vi "Test Bench.vi"() -> ()   [LabVIEW 2018, in "TwinCAT ADS.lvclass"]
uses:
  TwinCAT ADS.lvclass
  Controls/Symbol Information.ctl
  Controls/PLC Type.ctl
  TwinCAT.Ads
panel:
  out "data string":string
  out "output array":u8[](array[numeric])
  out "Value":variant
  out "PLC Type":T1
  out "IsStruct":bool
  out "Symbol Information":T2 {"Type ID" items=["ADST_VOID"=0, "ADST_INT16"=2, "ADST_INT32"=3, "ADST_REAL32"=4, "ADST_REAL64"=5, "ADST_INT8"=16, "ADST_UINT8"=17, "ADST_UINT16"=18, "ADST_UINT32"=19, "ADST_INT64"=20, "ADST_UINT64"=21, "ADST_STRING"=30, "ADST_WSTRING"=31, "ADST_REAL80"=32, "ADST_BIT"=33, "ADST_MAXTYPES"=34, "ADST_BIGTYPE"=65]; "Type Category" items=["Unknown, None"=0, "Primitive"=1, "Alias"=2, "Enum"=3, "Array"=4, "Struct"=5, "FunctionBlock"=6, "Program"=7, "Function"=8, "SubRange"=9, "String"=10, "Bitset"=12, "Pointer"=13, "Union"=14, "Reference"=15, "Interface"=16]}
  out "Out Params":variant[](array[variant])
  out "Return":variant
  out "x-y":dbl format="%^#_6e"
  out "*(type *) &x":u8[](array[numeric])
  out "Byte Stream":u8[](array[numeric])
  # "21.7E-6"
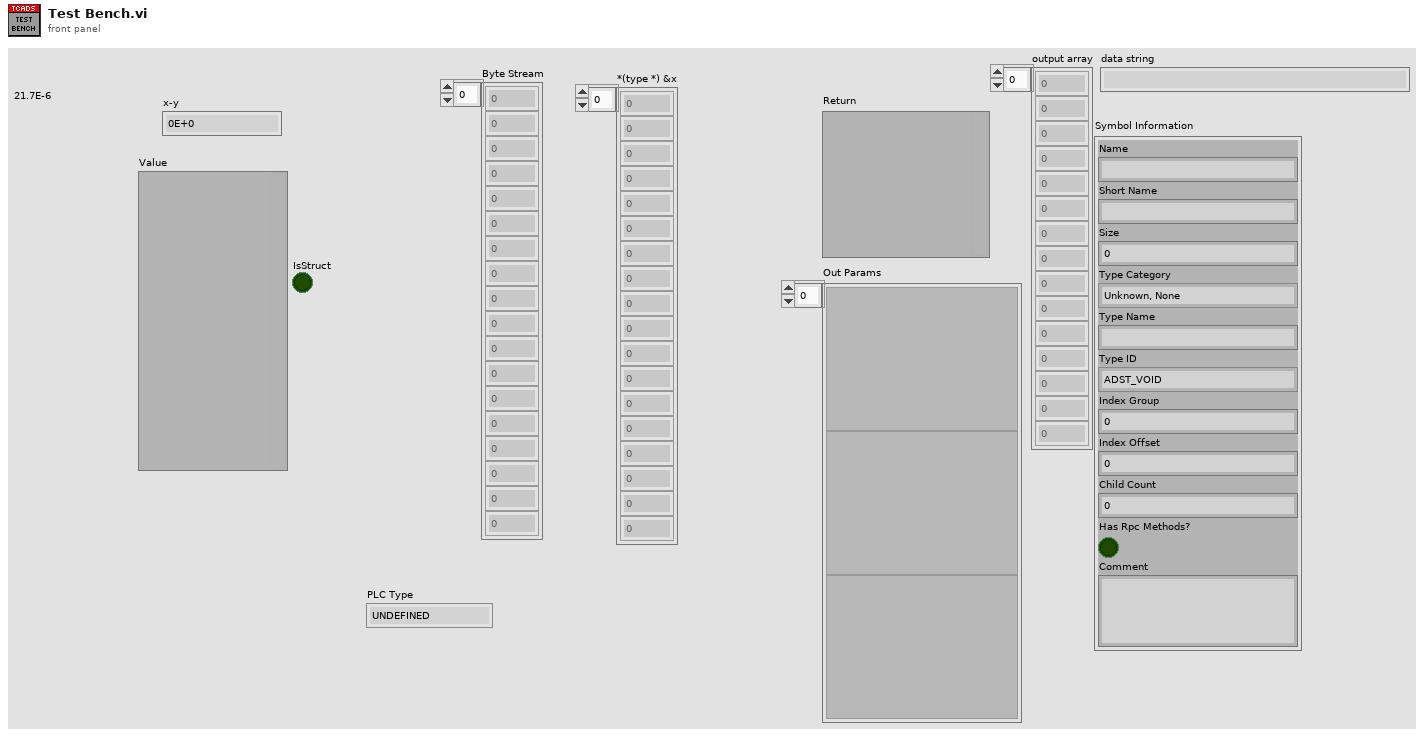
[diagram p1: front panel]
types:
  T1 = typedef "TwinCAT ADS.lvclass/PLC Type.ctl" = enum16{"UNDEFINED", "INT", "DINT", "REAL", "LREAL", "SINT", "BYTE", "UINT", "UDINT", "LINT", "ULINT", "STRING", "WSTRING", "BOOL", "TIME", "LTIME", "DATE", "DT", "TOD", "ARRAY", "JAGGED ARRAY", "STRUCT", "FUNCTION BLOCK", "UNION", "POINTER", "USER DEFINED"}
  T2 = typedef "TwinCAT ADS.lvclass/Symbol Information.ctl" = cluster{"Name":string, "Short Name":string, "Size":i32, "Type Category":i32, "Type Name":string, "Type ID":i32, "Index Group":i64, "Index Offset":i64, "Child Count":i32, "Has Rpc Methods?":bool, "Comment":string}
  T3 = enum16{"big-endian, network order", "native, host order", "little-endian"}
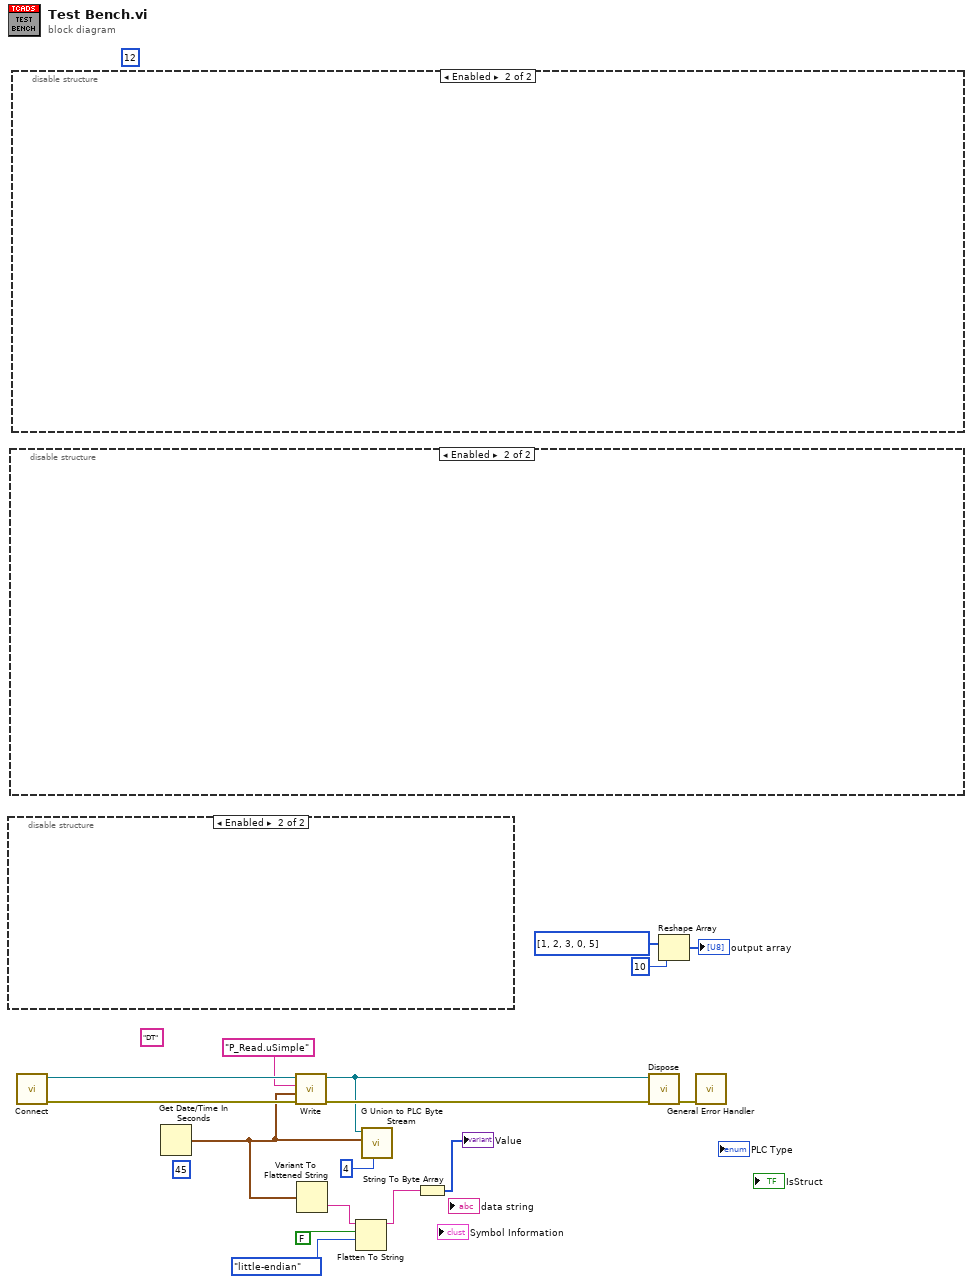
[diagram p0: block diagram]
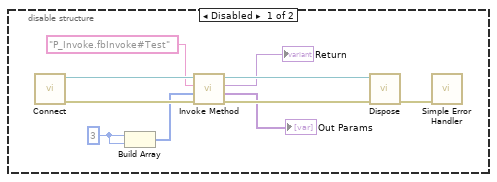
[diagram p2: hidden frame]
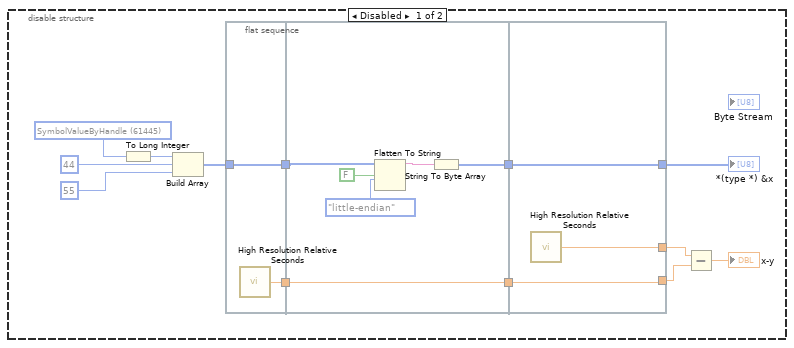
[diagram p3: hidden frame]
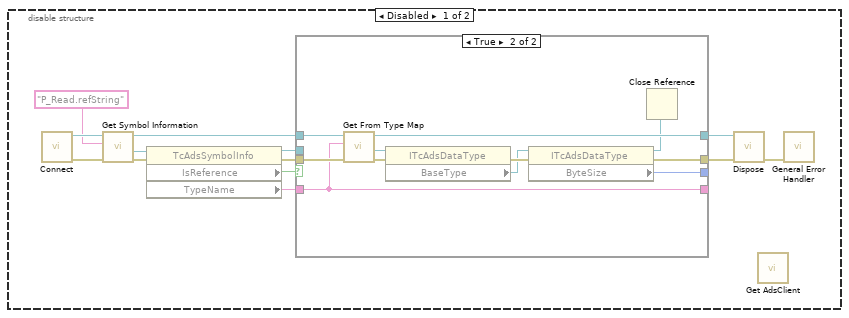
[diagram p4: hidden frame]
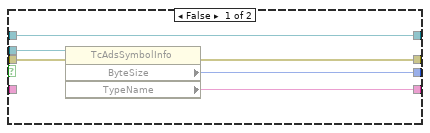
[diagram p5: hidden frame]
diagram:
  (unwired) u8 45 ("new element/subarray")
  (unwired) "DT" ("Type Name")
  (unwired) i16 12
  n1 = disable-structure shown="Enabled" {
    frame Disabled {
      w17 = 3
      n2 = call "Connect.vi"() -> ("error out"=w24:errorcluster, "TwinCAT ADS out"=w25:refnum<class "TwinCAT ADS.lvclass">)  [unwired: 10 in]
      n3 = Build Array(w17, w17) -> (w18:i32[])
      n4 = call "Invoke Method.vi"("error in (no error)"=w24, "In Parameters"=w18, "Function Block#Method"="P_Invoke.fbInvoke#Test", "TwinCAT ADS in"=w25) -> ("error out"=w23:errorcluster, "Out Parameters"=→"Out Params":variant[], "Return"=→"Return":variant, "TwinCAT ADS out"=w22:refnum<class "TwinCAT ADS.lvclass">)  [unwired: 4 in]
      n5 = call "Dispose.vi"("error in (no error)"=w23, "TwinCAT ADS in"=w22) -> ("error out"=w26:errorcluster)  [unwired: 9 in]
      n6 = call <vilib>:"Simple Error Handler.vi"("error in (no error)"=w26) -> ()  [unwired: 4 in, 5 out]
    }
    frame Enabled {
    }
  }
  n7 = disable-structure shown="Enabled" {
    frame Disabled {
      w32 = u32 61445 items=["PlcRWIB"=16384, "PlcRWOB"=16400, "PlcRWMB"=16416, "PlcRWRB"=16432, "PlcRWDB"=16448, "SymbolTable"=61440, "SymbolName"=61441, "SymbolValue"=61442, "SymbolHandleByName"=61443, "SymbolValueByName"=61444, "SymbolValueByHandle"=61445, "SymbolReleaseHandle"=61446, "SymbolInfoByName"=61447, "SymbolVersion"=61448, "SymbolInfoByNameEx"=61449, "SymbolDownload"=61450, "SymbolUpload"=61451, "SymbolUploadInfo"=61452, "SymbolNote"=61456, "IOImageRWIB"=61472, "IOImageRWIX"=61473, "IOImageRWOB"=61488, "IOImageRWOX"=61489, "IOImageClearI"=61504, "IOImageClearO"=61520, "SumCommandRead"=61568, "SumCommandWrite"=61569, "SumCommandReadWrite"=61570, "SumCommandReadEx"=61571, "SumCommandReadEx2"=61572, "SumCommandAddDevNote"=61573, "SumCommandDelDevNote"=61574, "DeviceData"=61696] ("SumCommandRead")
      n8 = To Long Integer(number=w32) -> (32bit integer=w33:i32)
      n9 = Build Array(w33, 44 ("Handle"), 55 ("ByteSize")) -> (w31:i32[])
      n10 = flat-sequence {
        tunnel: w31 -> [w41]
        tunnel: [w41] -> w39
        tunnel: [w40] -> w38
        tunnel: w39 -> [w44]
        tunnel: [w42] -> w37
        tunnel: w38 -> [w47]
        tunnel: [w47] -> w36
        tunnel: [w50] -> w27
        tunnel: w37 -> [w50]
        tunnel: w36 -> [w49]
        tunnel: [w49] -> w29
        tunnel: [w48] -> w30
        frame #0 {
          n11 = call <vilib>:"High Resolution Relative Seconds.vi"() -> ("relative seconds"=w40:dbl)
        }
        frame #1 {
          n12 = Flatten To String(anything=w44, prepend array or string size? (T)=FALSE, byte order (0:big-endian, network order)=T3."little-endian" ("Byte Order (little-endian)")) -> (data string=w43:string)  [unwired: 1 in, 2 out]
          n13 = String To Byte Array(string=w43) -> (unsigned byte array=w42:u8[])
        }
        frame #2 {
          n14 = call <vilib>:"High Resolution Relative Seconds.vi"() -> ("relative seconds"=w48:dbl)
        }
      }
      n15 = Subtract(x=w30, y=w29) -> (x-y=→"x-y":dbl)
      "*(type *) &x" <- w27
    }
    frame Enabled {
    }
  }
  n16 = disable-structure shown="Enabled" {
    frame Disabled {
      n17 = call "Connect.vi"() -> ("error out"=w59:errorcluster, "TwinCAT ADS out"=w60:refnum<class "TwinCAT ADS.lvclass">)  [unwired: 10 in]
      n18 = call "Get Symbol Information.vi"("error in (no error)"=w59, "Symbol Name"="P_Read.refString", "TwinCAT ADS in"=w60) -> ("error out"=w62:errorcluster, ".NET Symbol Information"=w61:refnum<k24>, "TwinCAT ADS out"=w56:refnum<class "TwinCAT ADS.lvclass">)  [unwired: 6 in]
      n19 = property class="TcAdsSymbolInfo"(reference=w61, error in=w62) -> (reference out=w51:refnum<k24>, error out=w55:errorcluster, "IsReference"=w57:bool, "TypeName"=w53:string)
      n20 = case shown="True" w57 {
        tunnel: w56 -> [w69 w80]
        tunnel: w55 -> [w68 w79]
        tunnel: [w69 w75] -> w54
        tunnel: w53 -> [_ w76]
        tunnel: [w64 w76] -> _
        tunnel: [w65 w72] -> _
        tunnel: [w66 w70] -> w52
        tunnel: w51 -> [w67 _]
        frame False {
          n21 = property class="TcAdsSymbolInfo"(reference=w67, error in=w68) -> (error out=w66:errorcluster, "ByteSize"=w65:i32, "TypeName"=w64:string)  [unwired: 1 out]
        }
        frame True {
          n22 = call "Get From Type Map.vi"("error in (no error)"=w79, "Type Name"=w76, "TwinCAT ADS in"=w80) -> ("error out"=w78:errorcluster, ".NET AdsDataType"=w77:refnum<k24>, "TwinCAT ADS out"=w75:refnum<class "TwinCAT ADS.lvclass">)  [unwired: 6 in]
          n23 = property class="ITcAdsDataType"(reference=w77, error in=w78) -> (error out=w74:errorcluster, "BaseType"=w73:refnum<k24>)  [unwired: 1 out]
          n24 = property class="ITcAdsDataType"(reference=w73, error in=w74) -> (reference out=w71:refnum<k24>, error out=w70:errorcluster, "ByteSize"=w72:i32)
          n25 = Close Reference(reference=w71) -> ()  [unwired: 1 in, 1 out]
        }
      }
      n26 = call "Dispose.vi"("error in (no error)"=w52, "TwinCAT ADS in"=w54) -> ("error out"=w63:errorcluster)  [unwired: 9 in]
      n27 = call "Get AdsClient.vi"() -> ()  [unwired: 9 in, 3 out]
      n28 = call <vilib>:"General Error Handler.vi"("error in (no error)"=w63) -> ()  [unwired: 10 in, 5 out]
    }
    frame Enabled {
    }
  }
  n29 = call "Connect.vi"() -> ("error out"=w12:errorcluster, "TwinCAT ADS out"=w11:refnum<class "TwinCAT ADS.lvclass">)  [unwired: 10 in]
  n30 = Get Date/Time In Seconds() -> (seconds since 1Jan1904=w3:timestamp)
  n31 = call "Write.vi"("error in (no error)"=w12, "Value"=w3, "Symbol Name"="P_Read.uSimple", "TwinCAT ADS in"=w11) -> ("error out"=w10:errorcluster, "TwinCAT ADS out"=w7:refnum<class "TwinCAT ADS.lvclass">)  [unwired: 6 in]
  n32 = Variant To Flattened String(Variant=w3) -> (data string=w5:string)  [unwired: 1 out]
  n33 = Flatten To String(anything=w5, prepend array or string size? (T)=FALSE, byte order (0:big-endian, network order)=T3."little-endian") -> (data string=w2:string)  [unwired: 1 in, 2 out]
  n34 = call "G Union to PLC Byte Stream.vi"("Byte Length"=4, "Value"=w3, "TwinCAT ADS in"=w7) -> ()  [unwired: 6 in, 3 out]
  n35 = String To Byte Array(string=w2) -> (unsigned byte array=→"Value":u8[])
  n36 = call "Dispose.vi"("error in (no error)"=w10, "TwinCAT ADS in"=w7) -> ("error out"=w16:errorcluster)  [unwired: 9 in]
  n37 = Reshape Array(u8[] [1, 2, 3, 0, 5] ("array"), 10 ("dimension size")) -> (→"output array":u8[])
  n38 = call <vilib>:"General Error Handler.vi"("error in (no error)"=w16) -> ()  [unwired: 10 in, 5 out]
